vi "DropVI_MQTT Server_withDebugTerminal.vi"() -> ()   [LabVIEW 2013]
uses:
  <vilib>/LabVIEW Open Source Project/Connection/Connection/Connection.lvclass
  Server class/Server.lvclass/Server.ctl
  Server class/Server.lvclass
  <vilib>/LabVIEW Open Source Project/MQTT Connection/MQTT_Base/Base Class/MQTT_Base.lvclass
  <vilib>/LabVIEW Open Source Project/Connection/Connection.TCP/Connection.TCP.lvclass
panel:
  out "error server":errorcluster
  out "NbConnections":u32
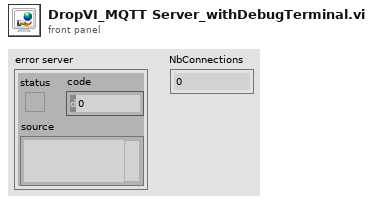
[diagram p1: front panel]
types:
  T1 = typedef "MQTT Server.lvlib/Server.lvclass/Public Events -- cluster.ctl" = cluster{"NbConnections":refnum<user-event>, "Client Event":refnum<user-event>}
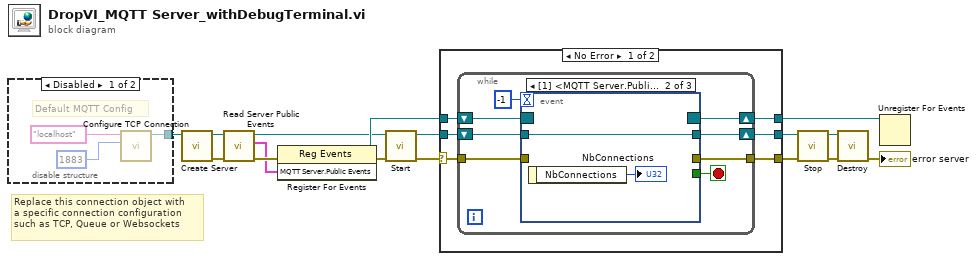
[diagram p0: block diagram]
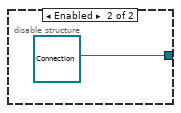
[diagram p2: hidden frame]
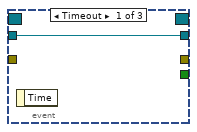
[diagram p3: hidden frame]
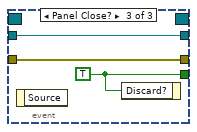
[diagram p4: hidden frame]
diagram:
  # "Replace this connection object with\na specific connection configuration\nsuch as TCP, Queue or Websockets"
  n1 = disable-structure shown="Disabled" {
    disable-tunnel: [w17 refnum<class "Connection.lvclass"> refnum ("Connection in")] -> w1
    frame Disabled {
      # "Default MQTT Config"
      n2 = call <vilib>:"Configure TCP Connection.vi"("remote port (80)"=u16 1883, "address (localhost)"="localhost") -> ("Connection.TCP"=w17:refnum<class "Connection.TCP.lvclass">)  [unwired: 8 in, 1 out]
    }
    frame Enabled {
    }
  }
  n3 = call "Create Server.vi"("Connection Configuration"=w1) -> ("error out"=w15:errorcluster, "Server"=w16:refnum<class "Server.lvclass">)  [unwired: 9 in]
  n4 = call "Read Server Public Events.vi"("error in (no error)"=w15, "Server in"=w16) -> ("error out"=w14:errorcluster, "MQTT Server.Public Events"=w13:T1, "Server out"=w10:refnum<class "Server.lvclass">)  [unwired: 7 in]
  n5 = register-events(error in=w14, w13) -> (reference out=w12:refnum<event-registration>, error out=w8:errorcluster)  [unwired: 1 in]
  n6 = call <vilib>:"Start.vi"("error in (no error)"=w8, "MQTT_Base in"=w10) -> ("error out"=w7:errorcluster, "MQTT_Base out"=w9:refnum<class "Server.lvclass">)  [unwired: 7 in, 1 out]
  n7 = case shown="No Error" w7 {
    selector: w7 -> [w21 w41]
    tunnel: w9 -> [w26 w43]
    tunnel: [w25 w43] -> w4
    tunnel: w12 -> [w24 w42]
    tunnel: [w23 w42] -> w11
    tunnel: [w22 w41] -> w2
    frame No Error {
      n8 = while {
        shift-right: [w31] -> w25
        shift-left: w26 -> [w33]
        tunnel: [w28] -> w22
        tunnel: w21 -> [w27]
        shift-right: [w29] -> w23
        shift-left: w24 -> [w30]
        stop <- w32 stop-if-true
        n9 = event shown="[1] <MQTT Server.Public Events.NbConnections>: User Event" {
          selector: w30 -> [_ _ _]
          dyn-events: [_ _ _] -> w29
          timeout: -1 -> [_ _ _]
          tunnel: w33 -> [w35 w37 w40]
          tunnel: [_ _ w38] -> w32
          tunnel: [w35 w37 w40] -> w31
          tunnel: [_ _ w39] -> w28
          tunnel: w27 -> [_ _ w39]
          event Timeout {
            n10 = event-data() -> ()  [unwired: 1 in, 1 out]
          }
          event User Event {
            n11 = event-data() -> ("NbConnections"=→"NbConnections":u32)  [unwired: 1 in]
          }
          event Panel Close? {
            w38 = TRUE ("Discard?")
            n12 = event-data() -> ()  [unwired: 1 in, 1 out]
            n13 = event-data("Discard?"=w38) -> ()  [unwired: 1 in, 1 out]
          }
        }
      }
    }
    frame Error {
    }
  }
  n14 = call <vilib>:"Stop.vi"("error in (no error)"=w2, "MQTT_Base in"=w4) -> ("error out"=w3:errorcluster, "MQTT_Base out"=w5:refnum<class "Server.lvclass">)  [unwired: 7 in, 1 out]
  n15 = call <vilib>:"Destroy.vi"("error in (no error)"=w3, "MQTT_Base in"=w5) -> ("error out"=→"error server":errorcluster)  [unwired: 8 in, 1 out]
  n16 = Unregister For Events(event registration refnum=w11) -> ()  [unwired: 1 in, 1 out]
